vi "Second step heating with process.vi"(0 "Arduino Resource In":T1={"VISA resource"="", "Board Type"=enum."Uno", "Connection Type"=enum."USB / Serial", "Bytes Per Packet (15)"=15}, 11 "Error In":errorcluster) -> (4 "Arduino Resource Out":T1={"VISA resource"="", "Board Type"=enum."Uno", "Connection Type"=enum."USB / Serial", "Bytes Per Packet (15)"=15}, 8 "isWork":bool, 15 "Error Out":errorcluster)   [LabVIEW 2016]
uses:
  <vilib>/LabVIEW Interface for Arduino/Type Defs/Arduino Resource.ctl
  <vilib>/LabVIEW Interface for Arduino/Type Defs/Board Type.ctl
  <vilib>/LabVIEW Interface for Arduino/LabVIEW Interface for Arduino.lvlib
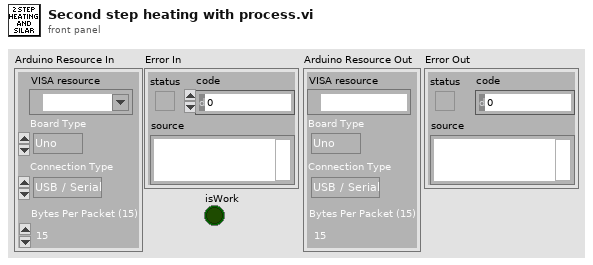
[diagram p1: front panel]
types:
  T1 = typedef "LabVIEW Interface for Arduino.lvlib/Arduino Resource.ctl" = cluster{"VISA resource":refnum<visa-resource-name>, "Board Type":T2, "Connection Type":enum8{"USB / Serial"}, "Bytes Per Packet (15)":u8}
  T2 = typedef "LabVIEW Interface for Arduino.lvlib/Board Type.ctl" = enum16{"Uno", "Dimuelanove w/Atmega 328", "Mega 2560"}
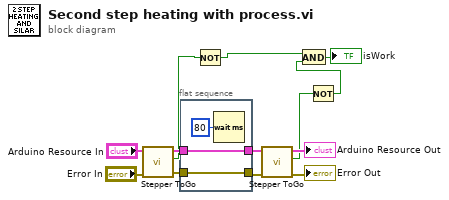
[diagram p0: block diagram]
diagram:
  n1 = call <vilib>:"Stepper ToGo.vi"("error in"="Error In", "Arduino Resource"="Arduino Resource In") -> ("error out"=w12:errorcluster, "Steps Remaining?"=w4:bool, "Arduino Resource Out"=w13:T1)  [unwired: 6 in, 1 out]
  n2 = flat-sequence {
    tunnel: w13 -> [w15]
    tunnel: [w15] -> w11
    tunnel: [w14] -> w10
    tunnel: w12 -> [w14]
    frame #0 {
      n3 = Wait (ms)(milliseconds to wait=u32 80) -> ()  [unwired: 1 out]
    }
  }
  n4 = Not(x=w4) -> (.not. x?=w3:bool)
  n5 = call <vilib>:"Stepper ToGo.vi"("error in"=w10, "Arduino Resource"=w11) -> ("error out"=→"Error Out":errorcluster, "Steps Remaining?"=w1:bool, "Arduino Resource Out"=→"Arduino Resource Out":T1)  [unwired: 6 in, 1 out]
  n6 = Not(x=w1) -> (.not. x?=w2:bool)
  n7 = And(x=w3, y=w2) -> (x .and. y?=→"isWork":bool)
